vi "Create LogMeasData Q.vi"(8 "error in (no error)":errorcluster, 10 "MeasData":T1, 11 "QName":string) -> (0 "error out":errorcluster, 3 "LogMeasDataQRef":refnum<queue>)   [LabVIEW 2017]
doc: "Developed by Kevin Thompson\nThompson Engineering, LLC\nkevin@thompsonengineering.net"
uses:
  TD MeasData--cluster.ctl
  GBL DataQ Ref.vi
panel:
  out "data reference":u32
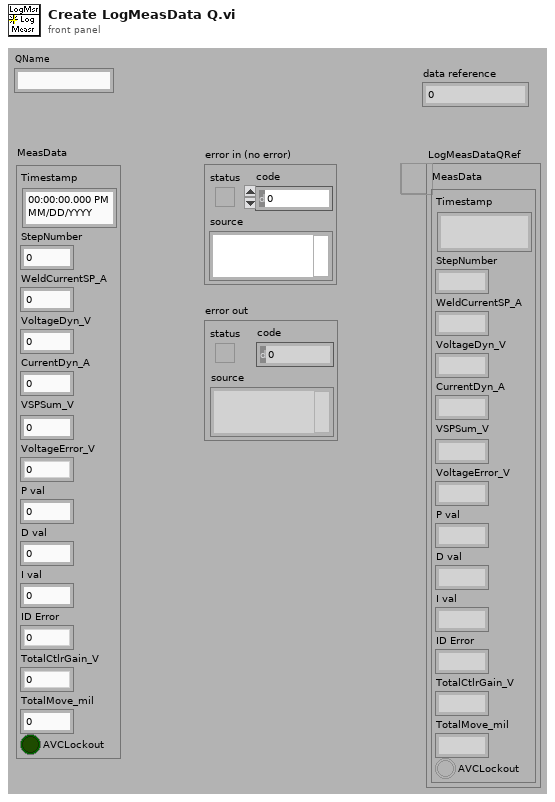
[diagram p1: front panel]
types:
  T1 = typedef "TD MeasData--cluster.ctl" = cluster{"Timestamp":timestamp, "StepNumber":i32, "WeldCurrentSP_A":dbl, "VoltageDyn_V":dbl, "CurrentDyn_A":dbl, "VSPSum_V":dbl, "VoltageError_V":dbl, "P val":dbl, "D val":dbl, "I val":dbl, "ID Error":dbl, "TotalCtlrGain_V":dbl, "TotalMove_mil":dbl, "AVCLockout":bool}
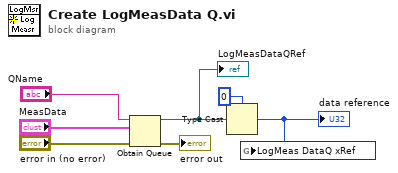
[diagram p0: block diagram]
diagram:
  n1 = Obtain Queue(name (unnamed)="QName", element data type="MeasData", error in (no error)="error in (no error)") -> (queue out=w1:refnum<queue>, error out=→"error out":errorcluster)  [unwired: 2 in, 1 out]
  "LogMeasDataQRef" <- w1
  n2 = Type Cast(type=u32 0, x=w1) -> (*(type *) &x=w3:u32)
  "data reference" <- w3
  n3 = global write "GBL DataQ Ref.vi" "LogMeas DataQ xRef"(w3) -> ()
